vi "EnableButtons.vi"(7 "Change Visibility?":bool, 8 "Error In":errorcluster, 9 "Enable?":bool, 11 "Button Ref Array":refnum<vi>[](array[refnum])) -> (0 "Error Out":errorcluster)   [LabVIEW 2020]
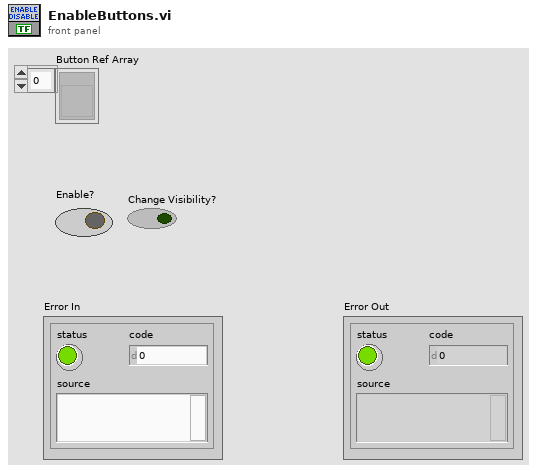
[diagram p1: front panel]
types:
  T1 = enum8{"Enabled", "Disabled", "Disabled and Grayed Out"}
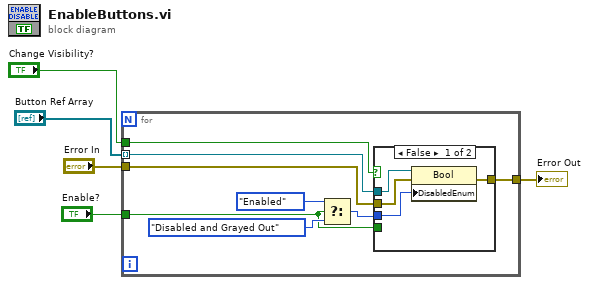
[diagram p0: block diagram]
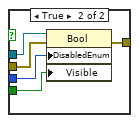
[diagram p2: hidden frame]
diagram:
  n1 = for {
    tunnel: "Button Ref Array" -> [w13] mode=indexing
    tunnel: "Enable?" -> [w6]
    tunnel: "Error In" -> [w9]
    tunnel: [w8] -> w2
    tunnel: "Change Visibility?" -> [w7]
    n2 = Select(t=T1."Enabled" ("Disabled"), s=w6, f=T1."Disabled and Grayed Out") -> (s? t:f=w11:T1)
    n3 = case shown="False" w7 {
      tunnel: w13 -> [w17 w22]
      tunnel: w11 -> [w15 w21]
      tunnel: w9 -> [w16 w20]
      tunnel: [w14 w19] -> w8
      tunnel: w6 -> [_ w18]
      frame False {
        n4 = property on="Property Node" class="Bool"(reference=w17, error in=w16, "DisabledEnum"=w15) -> (error out=w14:errorcluster)  [unwired: 1 out]
      }
      frame True {
        n5 = property on="Property Node" class="Bool"(reference=w22, error in=w20, "DisabledEnum"=w21, "Visible"=w18) -> (error out=w19:errorcluster)  [unwired: 1 out]
      }
    }
  }
  "Error Out" <- w2
